vi "Chirp2.vi"(9 "Chirp Parameters (in)":T1, 10 "DataPoints (in)":csg[](array[numeric]), 11 "Sub-band Sample Rate (in)":dbl) -> (3 "ChirpedData (out)":csg[](array[numeric]))   [LabVIEW 2015, in "SETI_LV.lvlib"]
uses:
  SETI_LV.lvlib
  TypeDefs/ChirpFFT Pairs.ctl
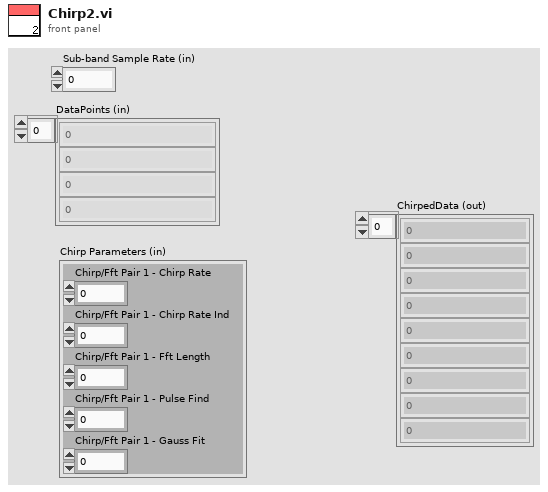
[diagram p1: front panel]
types:
  T1 = typedef "SETI_LV.lvlib/ChirpFFT Pairs.ctl" = cluster{"Chirp/Fft Pair 1 - Chirp Rate":dbl, "Chirp/Fft Pair 1 - Chirp Rate Ind":i32, "Chirp/Fft Pair 1 - Fft Length":i32, "Chirp/Fft Pair 1 - Pulse Find":i32, "Chirp/Fft Pair 1 - Gauss Fit":i32}
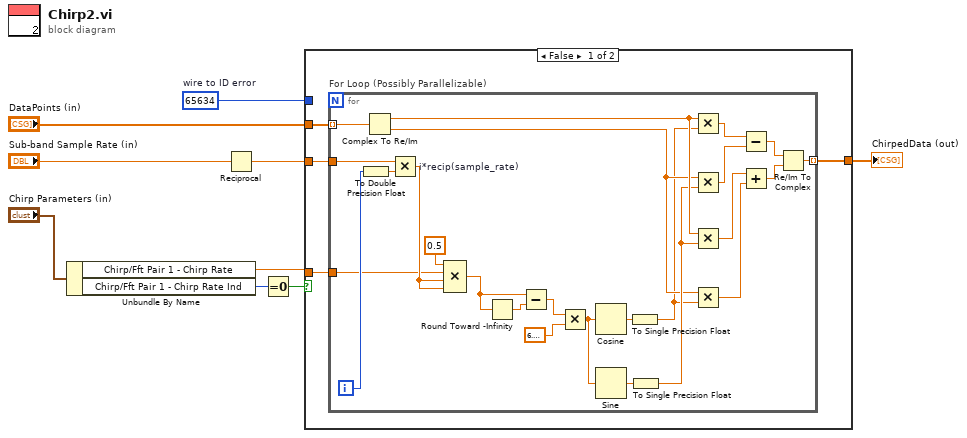
[diagram p0: block diagram]
diagram:
  w9 = 65634  # wire to ID error
  n1 = Unbundle By Name("Chirp Parameters (in)") -> ("Chirp/Fft Pair 1 - Chirp Rate"=w1:dbl, "Chirp/Fft Pair 1 - Chirp Rate Ind"=w3:i32)
  n2 = Reciprocal(x="Sub-band Sample Rate (in)") -> (1/x=w6:dbl)
  n3 = Equal To 0?(x=w3) -> (x = 0?=w8:bool)
  n4 = case shown="False" w8 {
    tunnel: "DataPoints (in)" -> [w13 w39]
    tunnel: [w10 w39] -> w7
    tunnel: w6 -> [w12 _]
    tunnel: w1 -> [w11 _]
    tunnel: w9 -> [_ _]
    frame False {
      n5 = for "For Loop (Possibly Parallelizable)" {
        tunnel: w13 -> [w38] mode=indexing
        tunnel: w12 -> [w37]
        tunnel: w11 -> [w32]
        tunnel: [w15] -> w10 mode=indexing
        i -> [w36]
        n6 = To Double Precision Float(number=w36) -> (double precision float=w35:dbl)
        n7 = Complex To Re/Im(x + iy=w38) -> (x=w19:sgl, y=w17:sgl)
        n8 = Multiply "i*recip(sample_rate)"(x=w37, y=w35) -> (x*y=w34:dbl)
        n9 = Compound Arithmetic op=MULTIPLY(0.5 ("value"), w32, w34, w34) -> (w31:dbl)
        n10 = Round Toward -Infinity(1:w31) -> (0:w30:dbl)
        n11 = Subtract(x=w31, y=w30) -> (x-y=w29:dbl)
        n12 = Multiply(x=w29, y=6.283185307179586) -> (x*y=w27:dbl)
        n13 = Cosine(x=w27) -> (cos(x)=w25:dbl)
        n14 = Sine(x=w27) -> (sin(x)=w26:dbl)
        n15 = To Single Precision Float(number=w25) -> (single precision float=w16:sgl)
        n16 = To Single Precision Float(number=w26) -> (single precision float=w18:sgl)
        n17 = Multiply(x=w19, y=w16) -> (x*y=w24:sgl)
        n18 = Multiply(x=w17, y=w18) -> (x*y=w23:sgl)
        n19 = Multiply(x=w19, y=w18) -> (x*y=w20:sgl)
        n20 = Multiply(x=w17, y=w16) -> (x*y=w21:sgl)
        n21 = Subtract(x=w24, y=w23) -> (x-y=w22:sgl)
        n22 = Add(x=w20, y=w21) -> (x+y=w14:sgl)
        n23 = Re/Im To Complex(1:w14, 2:w22) -> (0:w15:csg)
      }
    }
    frame True {
    }
  }
  "ChirpedData (out)" <- w7
